vi "last_array_row.vi"(1 "array":bool[][](array[boolean])) -> (0 "subarray":bool[](array[boolean]))   [LabVIEW 2013]
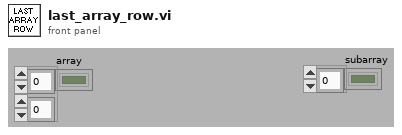
[diagram p1: front panel]
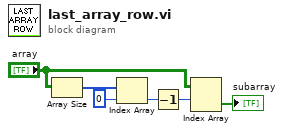
[diagram p0: block diagram]
diagram:
  n1 = Array Size(array="array") -> (size(s)=w5:i32[])
  n2 = Index Array(array=w5, index=0) -> (element=w2:i32)
  n3 = Decrement(x=w2) -> (x-1=w1:i32)
  n4 = Index Array(array="array", index (row)=w1) -> (element=→"subarray":bool[])  [unwired: 1 in]
